vi "WriteNdimArrayToCSV(SubVI).vi"(10 "Eightfold Path":path, 11 "N-dim Array":dbl[][](array[numeric])) -> ()   [LabVIEW 2017]
uses:
  <vilib>/Utility/file.llb/Write Delimited Spreadsheet (DBL).vi
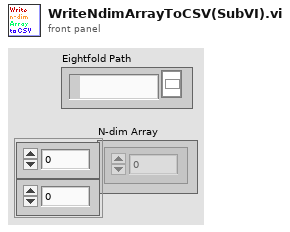
[diagram p1: front panel]
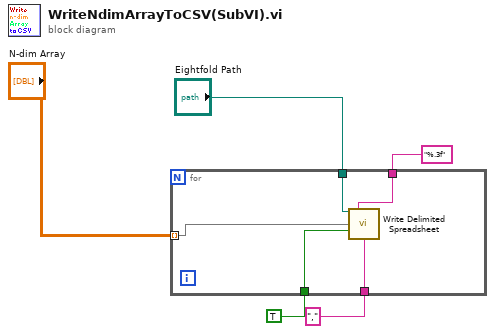
[diagram p0: block diagram]
diagram:
  n1 = for {
    tunnel: "N-dim Array" -> [w10] mode=indexing
    tunnel: "Eightfold Path" -> [w9]
    tunnel: "%.3f" -> [w8]
    tunnel: "," ("delimiter (\\t)") -> [w7]
    tunnel: TRUE ("append to file? (new file:F)") -> [w6]
    n2 = call-poly <vilib>:"Write Delimited Spreadsheet.vi"("file path (dialog if empty)"=w9, "format (%.3f)"=w8, "1D data"=w10, "append to file? (new file:F)"=w6, "delimiter (\\t)"=w7) -> ()  [unwired: 9 in, 2 out]
  }
